vi "CoerceLeftRight.vi"(9 "Left":dbl(slide) scale=1.0..-1.0, 10 "Forward":dbl(slide) scale=-1.0..1.0) -> (1 "Left":dbl(slide) scale=1.0..-1.0, 2 "Forward":dbl(slide) scale=-1.0..1.0)   [LabVIEW 2017]
panel:
  # "Input (percentage)"
  # "Out (after limiting)"
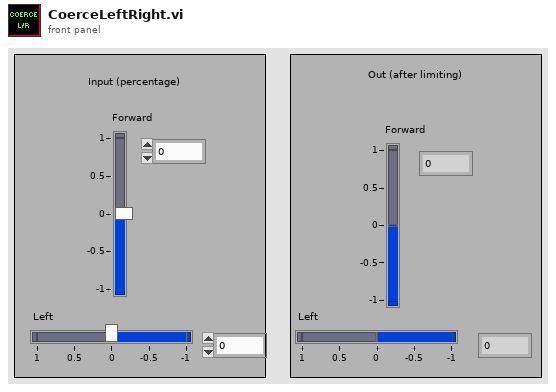
[diagram p1: front panel]
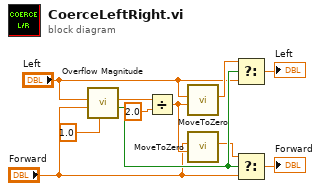
[diagram p0: block diagram]
diagram:
  n1 = call "Overflow Magnitude.vi"("Threshold"=1.0, "Input 2"="Forward", "Input 1"="Left") -> ("Overflow"=w9:bool, "Overflow Magnitude"=w11:dbl)  [unwired: 7 in]
  n2 = Divide(x=w11, y=2.0) -> (x/y=w7:dbl)
  n3 = call "MoveToZero.vi"("Decrease"=w7, "Value"="Left") -> ("Out"=w5:dbl)  [unwired: 9 in]
  n4 = call "MoveToZero.vi"("Decrease"=w7, "Value"="Forward") -> ("Out"=w6:dbl)  [unwired: 9 in]
  n5 = Select(t=w5, s=w9, f="Left") -> (s? t:f=→"Left":dbl)
  n6 = Select(t=w6, s=w9, f="Forward") -> (s? t:f=→"Forward":dbl)
